vi "Get Class Private Data.vi"(11 "Class":T1) -> (1 "Value":variant, 2 "Name":string, 3 "LVClassLibrary":refnum<vi>)   [LabVIEW 2018, in "LVClassByRef.lvlib"]
uses:
  <resource>/Framework/Providers/LVClassByRef/LVClassByRef.lvlib
  <resource>/Framework/Providers/API/ItemRef.ctl
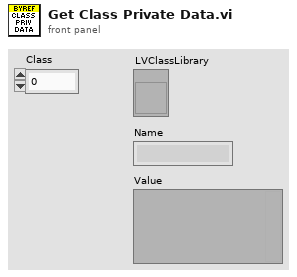
[diagram p1: front panel]
types:
  T1 = typedef "ItemRef.ctl" = u64
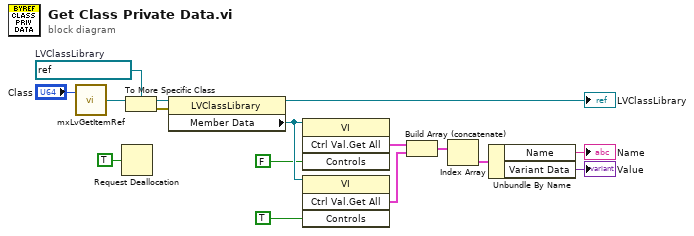
[diagram p0: block diagram]
diagram:
  w15 = refnum<vi> refnum  # LVClassLibrary
  n1 = call <resource>:"mxLvGetItemRef.vi"("Item"="Class") -> ("Item Refnum"=w16:refnum<vi>)  [unwired: 1 in, 2 out]
  n2 = Request Deallocation(TRUE ("flag")) -> ()
  n3 = To More Specific Class(target class=w15, reference=w16) -> (specific class reference=w14:refnum<vi>, error out=w13:errorcluster)  [unwired: 1 in]
  n4 = property class="LVClassLibrary"(reference=w14, error in=w13) -> (reference out=→"LVClassLibrary":refnum<vi>, "Member Data"=w11:refnum<vi>)  [unwired: 1 out]
  n5 = invoke class="VI" method="Ctrl Val.Get All"(reference=w11, "Controls"=FALSE) -> ("Get All Control Values Variant"=w12:cluster{"Name":string, "Variant Data":variant}[])  [unwired: 2 in, 3 out]
  n6 = invoke class="VI" method="Ctrl Val.Get All"(reference=w11, "Controls"=TRUE) -> ("Get All Control Values Variant"=w7:cluster{"Name":string, "Variant Data":variant}[])  [unwired: 2 in, 3 out]
  n7 = Build Array (concatenate)(w12, w7) -> (w8:cluster{"Name":string, "Variant Data":variant}[])
  n8 = Index Array(array=w8) -> (element=w6:cluster{"Name":string, "Variant Data":variant})  [unwired: 1 in]
  n9 = Unbundle By Name(w6) -> ("Name"=→"Name":string, "Variant Data"=→"Value":variant)
